vi "Wait for Operation Complete.vi"(8 "error in (no error)":errorcluster, 9 "Maximum Time (2000ms)":u32=2000, 11 "VISA resource name":refnum<visa-resource-name>) -> (0 "error out":errorcluster, 3 "VISA resource name out":refnum<visa-resource-name>)   [LabVIEW 2012]
doc: "Waits for the instrument to complete the execution of all pending operations."
panel:
  out "Numeric":i32
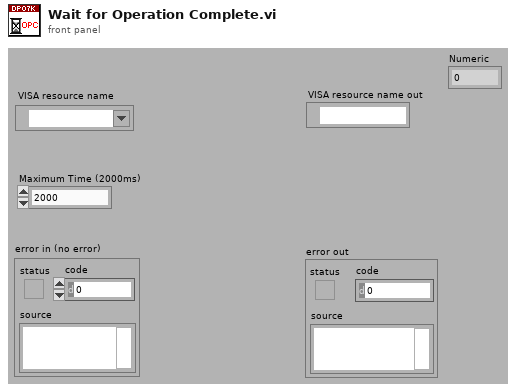
[diagram p1: front panel]
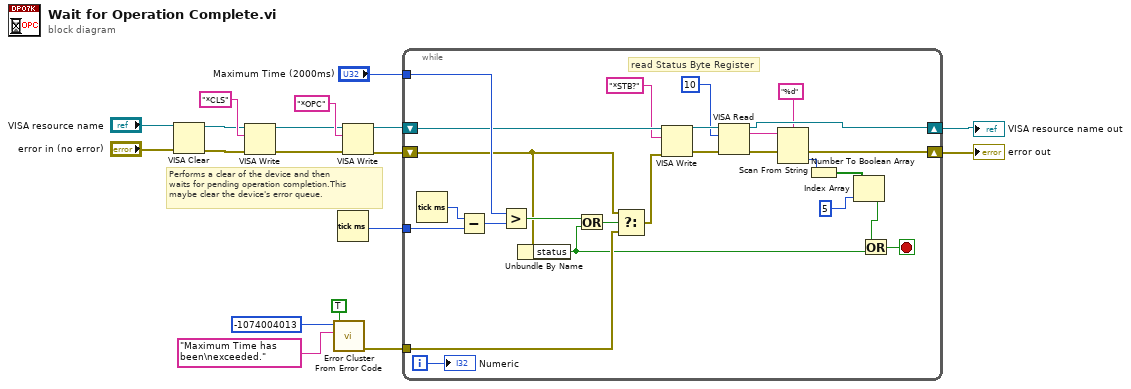
[diagram p0: block diagram]
diagram:
  # "Performs a clear of the device and then \nwaits for pending operation completion.This \nmaybe clear the device's error queue."
  n1 = VISA Clear(VISA resource name="VISA resource name", error in (no error)="error in (no error)") -> (VISA resource name out=w4:refnum<visa-resource-name>, error out=w3:errorcluster)
  n2 = VISA Write(VISA resource name=w4, write buffer="*CLS", error in (no error)=w3) -> (VISA resource name out=w2:refnum<visa-resource-name>, error out=w1:errorcluster)  [unwired: 1 out]
  n3 = call <vilib>:"Error Cluster From Error Code.vi"("show call chain? (False)"=TRUE, "error message (\"\")"="Maximum Time has been\nexceeded." ("error message (\"\")"), "error code (0)"=-1074004013) -> ("error out"=w8:errorcluster)  [unwired: 6 in]
  n4 = Tick Count (ms)() -> (millisecond timer value=w13:u32)
  n5 = VISA Write(VISA resource name=w2, write buffer="*OPC", error in (no error)=w1) -> (VISA resource name out=w15:refnum<visa-resource-name>, error out=w14:errorcluster)  [unwired: 1 out]
  n6 = while {
    tunnel: w13 -> [w41]
    tunnel: "Maximum Time (2000ms)" -> [w37]
    tunnel: w8 -> [w34]
    shift-right: [w24] -> w7
    shift-left: w15 -> [w31]
    shift-right: [w20] -> w6
    shift-left: w14 -> [w33]
    i -> [w19]
    stop <- w39 stop-if-true
    # "read Status Byte Register"
    n7 = Tick Count (ms)() -> (millisecond timer value=w42:u32)
    n8 = Subtract(x=w42, y=w41) -> (x-y=w38:u32)
    n9 = Greater?(x=w37, y=w38) -> (0:w36:bool)
    n10 = Unbundle By Name(w33) -> ("status"=w32:bool)
    n11 = Or(x=w36, y=w32) -> (x .or. y?=w35:bool)
    n12 = Select(t=w33, s=w35, f=w34) -> (s? t:f=w30:errorcluster)
    n13 = VISA Write(VISA resource name=w31, write buffer="*STB?", error in (no error)=w30) -> (VISA resource name out=w28:refnum<visa-resource-name>, error out=w27:errorcluster)  [unwired: 1 out]
    n14 = VISA Read(VISA resource name=w28, byte count=u32 10, error in (no error)=w27) -> (VISA resource name out=w24:refnum<visa-resource-name>, read buffer=w23:string, error out=w25:errorcluster)  [unwired: 1 out]
    n15 = Scan From String(format string="%d", input string=w23, error in=w25) -> (error out=w20:errorcluster, output 1=w21:i32)  [unwired: 2 in, 2 out]
    n16 = Number To Boolean Array(number=w21) -> (Boolean array=w44:bool[])
    n17 = Index Array(array=w44, index=5) -> (element=w40:bool)
    n18 = Or(x=w40, y=w32) -> (x .or. y?=w39:bool)
    "Numeric" <- w19
  }
  "VISA resource name out" <- w7
  "error out" <- w6
